vi "ParseSlaveRWw.vi"(1 "Node RWw":u16[][](array[numeric])) -> (0 "力觉力":sgl[](array[numeric]) format="%.2f")   [LabVIEW 2018]
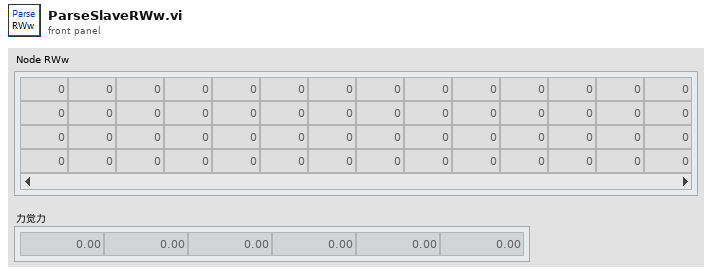
[diagram p1: front panel]
types:
  T1 = cluster{"当前泄漏量":sgl, "稳定泄漏量":sgl, "当前压力":sgl, "稳定压力":sgl, "风门闭电压":sgl, "风门开电压":sgl, "LED电流":sgl, "LED电压":sgl}
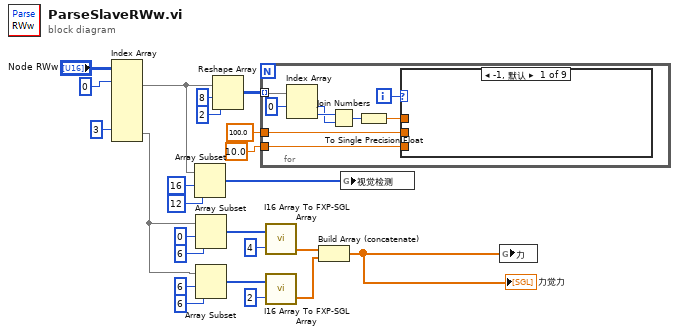
[diagram p0: block diagram]
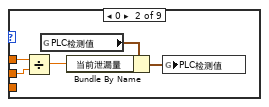
[diagram p2: hidden frame]
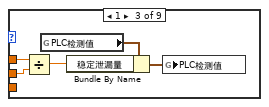
[diagram p3: hidden frame]
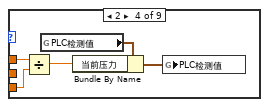
[diagram p4: hidden frame]
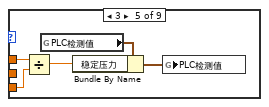
[diagram p5: hidden frame]
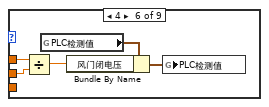
[diagram p6: hidden frame]
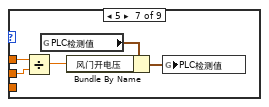
[diagram p7: hidden frame]
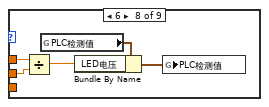
[diagram p8: hidden frame]
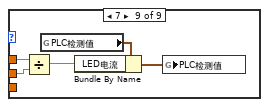
[diagram p9: hidden frame]
diagram:
  n1 = Index Array(array="Node RWw", index (row) #1=0 ("索引 (行)"), index (row) #4=3 ("索引 (行)")) -> (element #1=w17:u16[], element #4=w4:u16[])  [unwired: 6 in, 2 out]
  n2 = Array Subset(array=w17, index=16 ("索引"), length=12 ("长度")) -> (w14:u16[])
  n3 = Array Subset(array=w4, index=0 ("索引"), length=6 ("长度")) -> (w11:u16[])
  n4 = Array Subset(array=w4, index=6 ("索引"), length=6 ("长度")) -> (w6:u16[])
  n5 = Reshape Array(w17, 8 ("维数大小"), 2 ("维数大小")) -> (w20:u16[][])
  n6 = for {
    tunnel: w20 -> [w33] mode=indexing
    tunnel: sgl 100.0 -> [w27]
    tunnel: sgl 10.0 -> [w26]
    i -> [w25]
    n7 = Index Array(array=w33, index #1=0 ("索引")) -> (element #1=w30:u16, element #2=w31:u16)  [unwired: 1 in]
    n8 = Join Numbers(hi=w31, lo=w30) -> ((hi.lo)=w29:u32)
    n9 = To Single Precision Float(number=w29) -> (single precision float=w28:sgl)
    n10 = case shown="-1, 默认" w25 {
      tunnel: w28 -> [_ w38 w43 w48 w53 w58 w63 w68 w73]
      tunnel: w27 -> [_ w37 w42 _ _ w57 w62 w67 w69]
      tunnel: w26 -> [_ _ _ w44 w49 _ _ _ _]
      frame -1, Default {
      }
      frame 0 {
        n11 = Divide(x=w38, y=w37) -> (x/y=w36:sgl)
        n12 = global read "全局 1.vi" "PLC检测值"() -> (w34:T1)
        n13 = Bundle By Name(cluster=w34, "当前泄漏量"=w36) -> (w35:T1)
        n14 = global write "全局 1.vi" "PLC检测值"(w35) -> ()
      }
      frame 1 {
        n15 = Divide(x=w43, y=w42) -> (x/y=w41:sgl)
        n16 = global read "全局 1.vi" "PLC检测值"() -> (w39:T1)
        n17 = Bundle By Name(cluster=w39, "稳定泄漏量"=w41) -> (w40:T1)
        n18 = global write "全局 1.vi" "PLC检测值"(w40) -> ()
      }
      frame 2 {
        n19 = Divide(x=w48, y=w44) -> (x/y=w47:sgl)
        n20 = global read "全局 1.vi" "PLC检测值"() -> (w45:T1)
        n21 = Bundle By Name(cluster=w45, "当前压力"=w47) -> (w46:T1)
        n22 = global write "全局 1.vi" "PLC检测值"(w46) -> ()
      }
      frame 3 {
        n23 = Divide(x=w53, y=w49) -> (x/y=w52:sgl)
        n24 = global read "全局 1.vi" "PLC检测值"() -> (w50:T1)
        n25 = Bundle By Name(cluster=w50, "稳定压力"=w52) -> (w51:T1)
        n26 = global write "全局 1.vi" "PLC检测值"(w51) -> ()
      }
      frame 4 {
        n27 = Divide(x=w58, y=w57) -> (x/y=w56:sgl)
        n28 = global read "全局 1.vi" "PLC检测值"() -> (w54:T1)
        n29 = Bundle By Name(cluster=w54, "风门闭电压"=w56) -> (w55:T1)
        n30 = global write "全局 1.vi" "PLC检测值"(w55) -> ()
      }
      frame 5 {
        n31 = Divide(x=w63, y=w62) -> (x/y=w61:sgl)
        n32 = global read "全局 1.vi" "PLC检测值"() -> (w59:T1)
        n33 = Bundle By Name(cluster=w59, "风门开电压"=w61) -> (w60:T1)
        n34 = global write "全局 1.vi" "PLC检测值"(w60) -> ()
      }
      frame 6 {
        n35 = Divide(x=w68, y=w67) -> (x/y=w66:sgl)
        n36 = global read "全局 1.vi" "PLC检测值"() -> (w64:T1)
        n37 = Bundle By Name(cluster=w64, "LED电压"=w66) -> (w65:T1)
        n38 = global write "全局 1.vi" "PLC检测值"(w65) -> ()
      }
      frame 7 {
        n39 = Divide(x=w73, y=w69) -> (x/y=w72:sgl)
        n40 = global read "全局 1.vi" "PLC检测值"() -> (w70:T1)
        n41 = Bundle By Name(cluster=w70, "LED电流"=w72) -> (w71:T1)
        n42 = global write "全局 1.vi" "PLC检测值"(w71) -> ()
      }
    }
  }
  n43 = call "I16 Array To FXP-SGL Array.vi"("小数位数"=4, "I16 Array"=w11) -> ("SGL Array"=w3:sgl[])  [unwired: 1 out]
  n44 = call "I16 Array To FXP-SGL Array.vi"("小数位数"=2, "I16 Array"=w6) -> ("SGL Array"=w2:sgl[])  [unwired: 1 out]
  n45 = Build Array (concatenate)(w3, w2) -> (w1:sgl[])
  "力觉力" <- w1
  n46 = global write "全局 1.vi" "视觉检测"(w14) -> ()
  n47 = global write "全局 1.vi" "力"(w1) -> ()
